vi "FlatToRichniswitch_grpc_SetAttributeViInt32Request.vi"(5 "OutputClusterType":T1, 11 "InputCluster":T4) -> (3 "OutputCluster":T1)   [LabVIEW 2021, in "NI Switch_client.lvlib"]
uses:
  NI Switch_client.lvlib
  niswitch_grpc_SetAttributeViInt32Request_attribute_value_enum/niswitch_grpc_SetAttributeViInt32Request_attribute_value_enum.lvclass
  niswitch_grpc_NiSwitchAttribute.ctl
  nidevice_grpc_Session.ctl
  niswitch_grpc_SetAttributeViInt32Request.ctl
  niswitch_grpc_NiSwitchInt32AttributeValues.ctl
  nidevice_grpc_Session_Flat.ctl
  niswitch_grpc_SetAttributeViInt32Request_Flat.ctl
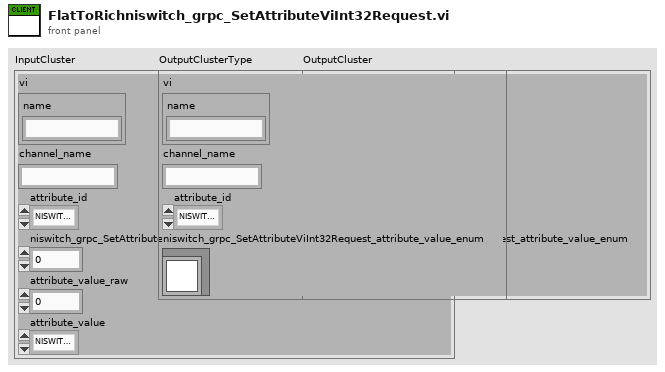
[diagram p1: front panel]
types:
  T1 = typedef "NI Switch_client.lvlib/niswitch_grpc_SetAttributeViInt32Request.ctl" = cluster{"vi":T2, "channel_name":string, "attribute_id":T3, "niswitch_grpc_SetAttributeViInt32Request_attribute_value_enum":refnum<class "niswitch_grpc_SetAttributeViInt32Request_attribute_value_enum.lvclass">}
  T2 = typedef "NI Switch_client.lvlib/nidevice_grpc_Session.ctl" = cluster{"name":string}
  T3 = typedef "NI Switch_client.lvlib/niswitch_grpc_NiSwitchAttribute.ctl" = enum32{"NISWITCH_ATTRIBUTE_UNSPECIFIED", "NISWITCH_ATTRIBUTE_RANGE_CHECK", "NISWITCH_ATTRIBUTE_QUERY_INSTRUMENT_STATUS", "NISWITCH_ATTRIBUTE_CACHE", "NISWITCH_ATTRIBUTE_SIMULATE", "NISWITCH_ATTRIBUTE_RECORD_COERCIONS", "NISWITCH_ATTRIBUTE_DRIVER_SETUP", "NISWITCH_ATTRIBUTE_INTERCHANGE_CHECK", "NISWITCH_ATTRIBUTE_CHANNEL_COUNT", "NISWITCH_ATTRIBUTE_SPECIFIC_DRIVER_PREFIX", "NISWITCH_ATTRIBUTE_IO_RESOURCE_DESCRIPTOR", "NISWITCH_ATTRIBUTE_LOGICAL_NAME", "NISWITCH_ATTRIBUTE_SUPPORTED_INSTRUMENT_MODELS", "NISWITCH_ATTRIBUTE_GROUP_CAPABILITIES", "NISWITCH_ATTRIBUTE_INSTRUMENT_FIRMWARE_REVISION", "NISWITCH_ATTRIBUTE_INSTRUMENT_MANUFACTURER", "NISWITCH_ATTRIBUTE_INSTRUMENT_MODEL", "NISWITCH_ATTRIBUTE_SPECIFIC_DRIVER_VENDOR", "NISWITCH_ATTRIBUTE_SPECIFIC_DRIVER_DESCRIPTION", "NISWITCH_ATTRIBUTE_SPECIFIC_DRIVER_CLASS_SPEC_MAJOR_VERSION", "NISWITCH_ATTRIBUTE_SPECIFIC_DRIVER_CLASS_SPEC_MINOR_VERSION", "NISWITCH_ATTRIBUTE_SPECIFIC_DRIVER_REVISION", "NISWITCH_ATTRIBUTE_SERIAL_NUMBER_I32", "NISWITCH_ATTRIBUTE_IS_WAITING_FOR_TRIG", "NISWITCH_ATTRIBUTE_TRIGGER_MODE", "NISWITCH_ATTRIBUTE_MASTER_SLAVE_TRIGGER_BUS", "NISWITCH_ATTRIBUTE_MASTER_SLAVE_SCAN_ADVANCED_BUS", "NISWITCH_ATTRIBUTE_CABLED_MODULE_TRIGGER_BUS", "NISWITCH_ATTRIBUTE_CABLED_MODULE_SCAN_ADVANCED_BUS", "NISWITCH_ATTRIBUTE_TRIGGER_INPUT_POLARITY", "NISWITCH_ATTRIBUTE_SCAN_ADVANCED_POLARITY", "NISWITCH_ATTRIBUTE_PARSED_SCAN_LIST", "NISWITCH_ATTRIBUTE_HANDSHAKING_INITIATION", "NISWITCH_ATTRIBUTE_NUMBER_OF_RELAYS", "NISWITCH_ATTRIBUTE_SERIAL_NUMBER", "NISWITCH_ATTRIBUTE_DIGITAL_FILTER_ENABLE", "NISWITCH_ATTRIBUTE_POWER_DOWN_LATCHING_RELAYS_AFTER_DEBOUNCE", "NISWITCH_ATTRIBUTE_ANALOG_BUS_SHARING_ENABLE", "NISWITCH_ATTRIBUTE_TEMPERATURE", "NISWITCH_ATTRIBUTE_IS_SOURCE_CHANNEL", "NISWITCH_ATTRIBUTE_IS_DEBOUNCED", "NISWITCH_ATTRIBUTE_IS_CONFIGURATION_CHANNEL", "NISWITCH_ATTRIBUTE_SETTLING_TIME", "NISWITCH_ATTRIBUTE_BANDWIDTH", "NISWITCH_ATTRIBUTE_MAX_DC_VOLTAGE", "NISWITCH_ATTRIBUTE_MAX_AC_VOLTAGE", "NISWITCH_ATTRIBUTE_MAX_SWITCHING_DC_CURRENT", "NISWITCH_ATTRIBUTE_MAX_SWITCHING_AC_CURRENT", "NISWITCH_ATTRIBUTE_MAX_CARRY_DC_CURRENT", "NISWITCH_ATTRIBUTE_MAX_CARRY_AC_CURRENT", "NISWITCH_ATTRIBUTE_MAX_SWITCHING_DC_POWER", "NISWITCH_ATTRIBUTE_MAX_SWITCHING_AC_POWER", "NISWITCH_ATTRIBUTE_MAX_CARRY_DC_POWER", "NISWITCH_ATTRIBUTE_MAX_CARRY_AC_POWER", "NISWITCH_ATTRIBUTE_CHARACTERISTIC_IMPEDANCE", "NISWITCH_ATTRIBUTE_WIRE_MODE", "NISWITCH_ATTRIBUTE_NUM_OF_ROWS", "NISWITCH_ATTRIBUTE_NUM_OF_COLUMNS", "NISWITCH_ATTRIBUTE_SCAN_LIST", "NISWITCH_ATTRIBUTE_SCAN_MODE", "NISWITCH_ATTRIBUTE_TRIGGER_INPUT", "NISWITCH_ATTRIBUTE_SCAN_ADVANCED_OUTPUT", "NISWITCH_ATTRIBUTE_IS_SCANNING", "NISWITCH_ATTRIBUTE_SCAN_DELAY", "NISWITCH_ATTRIBUTE_CONTINUOUS_SCAN"}
  T4 = typedef "NI Switch_client.lvlib/niswitch_grpc_SetAttributeViInt32Request_Flat.ctl" = cluster{"vi":T5, "channel_name":string, "attribute_id":T3, "niswitch_grpc_SetAttributeViInt32Request_attribute_value_enum_selected_index":i32, "attribute_value_raw":i32, "attribute_value":T6}
  T5 = typedef "NI Switch_client.lvlib/nidevice_grpc_Session_Flat.ctl" = cluster{"name":string}
  T6 = typedef "NI Switch_client.lvlib/niswitch_grpc_NiSwitchInt32AttributeValues.ctl" = enum32{"NISWITCH_INT32_UNSPECIFIED", "NISWITCH_INT32_HANDSHAKING_INITIATION_VAL_MEASUREMENT_DEVICE_INITIATED", "NISWITCH_INT32_HANDSHAKING_INITIATION_VAL_SWITCH_INITIATED", "NISWITCH_INT32_SCAN_ADVANCED_OUTPUT_VAL_NONE", "NISWITCH_INT32_SCAN_ADVANCED_OUTPUT_VAL_EXTERNAL", "NISWITCH_INT32_SCAN_ADVANCED_OUTPUT_VAL_TTL0", "NISWITCH_INT32_SCAN_ADVANCED_OUTPUT_VAL_TTL1", "NISWITCH_INT32_SCAN_ADVANCED_OUTPUT_VAL_TTL2", "NISWITCH_INT32_SCAN_ADVANCED_OUTPUT_VAL_TTL3", "NISWITCH_INT32_SCAN_ADVANCED_OUTPUT_VAL_TTL4", "NISWITCH_INT32_SCAN_ADVANCED_OUTPUT_VAL_TTL5", "NISWITCH_INT32_SCAN_ADVANCED_OUTPUT_VAL_TTL6", "NISWITCH_INT32_SCAN_ADVANCED_OUTPUT_VAL_TTL7", "NISWITCH_INT32_SCAN_ADVANCED_OUTPUT_VAL_PXI_STAR", "NISWITCH_INT32_SCAN_ADVANCED_OUTPUT_VAL_REARCONNECTOR", "NISWITCH_INT32_SCAN_ADVANCED_OUTPUT_VAL_FRONTCONNECTOR", "NISWITCH_INT32_SCAN_ADVANCED_OUTPUT_VAL_REARCONNECTOR_MODULE1", "NISWITCH_INT32_SCAN_ADVANCED_OUTPUT_VAL_REARCONNECTOR_MODULE2", "NISWITCH_INT32_SCAN_ADVANCED_OUTPUT_VAL_REARCONNECTOR_MODULE3", "NISWITCH_INT32_SCAN_ADVANCED_OUTPUT_VAL_REARCONNECTOR_MODULE4", "NISWITCH_INT32_SCAN_ADVANCED_OUTPUT_VAL_REARCONNECTOR_MODULE5", "NISWITCH_INT32_SCAN_ADVANCED_OUTPUT_VAL_REARCONNECTOR_MODULE6", "NISWITCH_INT32_SCAN_ADVANCED_OUTPUT_VAL_REARCONNECTOR_MODULE7", "NISWITCH_INT32_SCAN_ADVANCED_OUTPUT_VAL_REARCONNECTOR_MODULE8", "NISWITCH_INT32_SCAN_ADVANCED_OUTPUT_VAL_REARCONNECTOR_MODULE9", "NISWITCH_INT32_SCAN_ADVANCED_OUTPUT_VAL_REARCONNECTOR_MODULE10", "NISWITCH_INT32_SCAN_ADVANCED_OUTPUT_VAL_REARCONNECTOR_MODULE11", "NISWITCH_INT32_SCAN_ADVANCED_OUTPUT_VAL_REARCONNECTOR_MODULE12", "NISWITCH_INT32_SCAN_ADVANCED_OUTPUT_VAL_FRONTCONNECTOR_MODULE1", "NISWITCH_INT32_SCAN_ADVANCED_OUTPUT_VAL_FRONTCONNECTOR_MODULE2", "NISWITCH_INT32_SCAN_ADVANCED_OUTPUT_VAL_FRONTCONNECTOR_MODULE3", "NISWITCH_INT32_SCAN_ADVANCED_OUTPUT_VAL_FRONTCONNECTOR_MODULE4", "NISWITCH_INT32_SCAN_ADVANCED_OUTPUT_VAL_FRONTCONNECTOR_MODULE5", "NISWITCH_INT32_SCAN_ADVANCED_OUTPUT_VAL_FRONTCONNECTOR_MODULE6", "NISWITCH_INT32_SCAN_ADVANCED_OUTPUT_VAL_FRONTCONNECTOR_MODULE7", "NISWITCH_INT32_SCAN_ADVANCED_OUTPUT_VAL_FRONTCONNECTOR_MODULE8", "NISWITCH_INT32_SCAN_ADVANCED_OUTPUT_VAL_FRONTCONNECTOR_MODULE9", "NISWITCH_INT32_SCAN_ADVANCED_OUTPUT_VAL_FRONTCONNECTOR_MODULE10", "NISWITCH_INT32_SCAN_ADVANCED_OUTPUT_VAL_FRONTCONNECTOR_MODULE11", "NISWITCH_INT32_SCAN_ADVANCED_OUTPUT_VAL_FRONTCONNECTOR_MODULE12", "NISWITCH_INT32_SCAN_ADVANCED_POLARITY_VAL_RISING_EDGE", "NISWITCH_INT32_SCAN_ADVANCED_POLARITY_VAL_FALLING_EDGE", "NISWITCH_INT32_SCAN_MODE_VAL_NONE", "NISWITCH_INT32_SCAN_MODE_VAL_BREAK_BEFORE_MAKE", "NISWITCH_INT32_SCAN_MODE_VAL_BREAK_AFTER_MAKE", "NISWITCH_INT32_TRIGGER_INPUT_VAL_IMMEDIATE", "NISWITCH_INT32_TRIGGER_INPUT_VAL_EXTERNAL", "NISWITCH_INT32_TRIGGER_INPUT_VAL_SOFTWARE_TRIG", "NISWITCH_INT32_TRIGGER_INPUT_VAL_TTL0", "NISWITCH_INT32_TRIGGER_INPUT_VAL_TTL1", "NISWITCH_INT32_TRIGGER_INPUT_VAL_TTL2", "NISWITCH_INT32_TRIGGER_INPUT_VAL_TTL3", "NISWITCH_INT32_TRIGGER_INPUT_VAL_TTL4", "NISWITCH_INT32_TRIGGER_INPUT_VAL_TTL5", "NISWITCH_INT32_TRIGGER_INPUT_VAL_TTL6", "NISWITCH_INT32_TRIGGER_INPUT_VAL_TTL7", "NISWITCH_INT32_TRIGGER_INPUT_VAL_PXI_STAR", "NISWITCH_INT32_TRIGGER_INPUT_VAL_REARCONNECTOR", "NISWITCH_INT32_TRIGGER_INPUT_VAL_FRONTCONNECTOR", "NISWITCH_INT32_TRIGGER_INPUT_VAL_REARCONNECTOR_MODULE1", "NISWITCH_INT32_TRIGGER_INPUT_VAL_REARCONNECTOR_MODULE2", "NISWITCH_INT32_TRIGGER_INPUT_VAL_REARCONNECTOR_MODULE3", "NISWITCH_INT32_TRIGGER_INPUT_VAL_REARCONNECTOR_MODULE4", "NISWITCH_INT32_TRIGGER_INPUT_VAL_REARCONNECTOR_MODULE5", "NISWITCH_INT32_TRIGGER_INPUT_VAL_REARCONNECTOR_MODULE6", "NISWITCH_INT32_TRIGGER_INPUT_VAL_REARCONNECTOR_MODULE7", "NISWITCH_INT32_TRIGGER_INPUT_VAL_REARCONNECTOR_MODULE8", "NISWITCH_INT32_TRIGGER_INPUT_VAL_REARCONNECTOR_MODULE9", "NISWITCH_INT32_TRIGGER_INPUT_VAL_REARCONNECTOR_MODULE10", "NISWITCH_INT32_TRIGGER_INPUT_VAL_REARCONNECTOR_MODULE11", "NISWITCH_INT32_TRIGGER_INPUT_VAL_REARCONNECTOR_MODULE12", "NISWITCH_INT32_TRIGGER_INPUT_VAL_FRONTCONNECTOR_MODULE1", "NISWITCH_INT32_TRIGGER_INPUT_VAL_FRONTCONNECTOR_MODULE2", "NISWITCH_INT32_TRIGGER_INPUT_VAL_FRONTCONNECTOR_MODULE3", "NISWITCH_INT32_TRIGGER_INPUT_VAL_FRONTCONNECTOR_MODULE4", "NISWITCH_INT32_TRIGGER_INPUT_VAL_FRONTCONNECTOR_MODULE5", "NISWITCH_INT32_TRIGGER_INPUT_VAL_FRONTCONNECTOR_MODULE6", "NISWITCH_INT32_TRIGGER_INPUT_VAL_FRONTCONNECTOR_MODULE7", "NISWITCH_INT32_TRIGGER_INPUT_VAL_FRONTCONNECTOR_MODULE8", "NISWITCH_INT32_TRIGGER_INPUT_VAL_FRONTCONNECTOR_MODULE9", "NISWITCH_INT32_TRIGGER_INPUT_VAL_FRONTCONNECTOR_MODULE10", "NISWITCH_INT32_TRIGGER_INPUT_VAL_FRONTCONNECTOR_MODULE11", "NISWITCH_INT32_TRIGGER_INPUT_VAL_FRONTCONNECTOR_MODULE12", "NISWITCH_INT32_TRIGGER_INPUT_POLARITY_VAL_RISING_EDGE", "NISWITCH_INT32_TRIGGER_INPUT_POLARITY_VAL_FALLING_EDGE", "NISWITCH_INT32_WIRE_MODE_VAL_1_WIRE", "NISWITCH_INT32_WIRE_MODE_VAL_2_WIRE", "NISWITCH_INT32_WIRE_MODE_VAL_4_WIRE"}
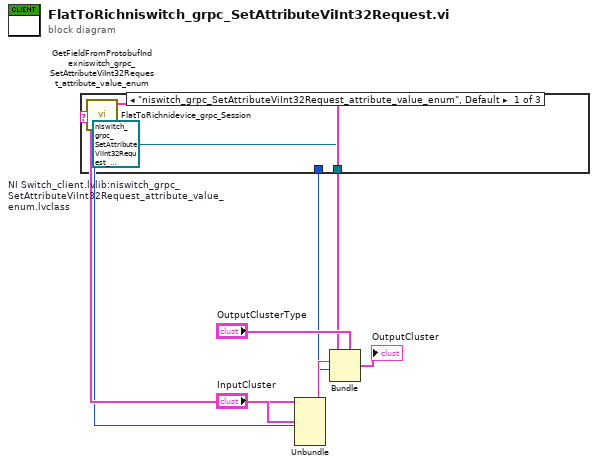
[diagram p0: block diagram]
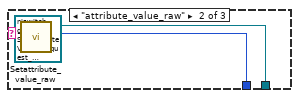
[diagram p2: hidden frame]
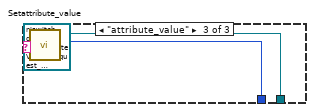
[diagram p3: hidden frame]
diagram:
  n1 = Unbundle "Unbundle"("InputCluster") -> ("vi"=w9:T5, "channel_name"=w7:string, "attribute_id"=w6:T3, "niswitch_grpc_SetAttributeViInt32Request_attribute_value_enum_selected_index"=w5:i32, "attribute_value_raw"=w2:i32, "attribute_value"=w1:T6)
  n2 = call "GetFieldFromProtobufIndexniswitch_grpc_SetAttributeViInt32Request_attribute_value_enum.vi"("protobuf index"=w5) -> ("oneof field name"=w4:string)
  n3 = case "niswitch_grpc_SetAttributeViInt32Request_attribute_value_enum" shown="\"niswitch_grpc_SetAttributeViInt32Request_attribute_value_enum\", Default" w4 {
    tunnel: [w13 w15 w18] -> w3
    tunnel: w2 -> [_ w16 _]
    tunnel: w1 -> [_ _ w19]
    frame "niswitch_grpc_SetAttributeViInt32Request_attribute_value_enum", Default {
      w13 = refnum<class "niswitch_grpc_SetAttributeViInt32Request_attribute_value_enum.lvclass"> refnum  # NI Switch_client.lvlib:niswitch_grpc_SetAttributeViInt32Request_attribute_value_enum.lvclass
    }
    frame "attribute_value_raw" {
      n4 = call "Setattribute_value_raw.vi"("Set_Val"=w16, "OneOfTemplate in"=refnum<class "niswitch_grpc_SetAttributeViInt32Request_attribute_value_enum.lvclass"> refnum) -> ("OneOfTemplate out"=w15:refnum<class "niswitch_grpc_SetAttributeViInt32Request_attribute_value_enum.lvclass">)  [unwired: 8 in, 1 out]
    }
    frame "attribute_value" {
      n5 = call "Setattribute_value.vi"("Set_Val"=w19, "OneOfTemplate in"=refnum<class "niswitch_grpc_SetAttributeViInt32Request_attribute_value_enum.lvclass"> refnum) -> ("OneOfTemplate out"=w18:refnum<class "niswitch_grpc_SetAttributeViInt32Request_attribute_value_enum.lvclass">)  [unwired: 8 in, 1 out]
    }
  }
  n6 = call "FlatToRichnidevice_grpc_Session.vi"("InputCluster"=w9) -> ("OutputCluster"=w8:T2)  [unwired: 10 in]
  n7 = Bundle "Bundle"(cluster="OutputClusterType", "vi"=w8, "channel_name"=w7, "attribute_id"=w6, "niswitch_grpc_SetAttributeViInt32Request_attribute_value_enum"=w3) -> (→"OutputCluster":T1)
